vi "Get All Open Projects.vi"(8 "error in (no error)":errorcluster) -> (0 "error out":errorcluster, 1 "Names":string[](array[string]), 3 "Project refs out":refnum<vi>[](array[refnum]))   [LabVIEW 2019, in "Configuration Tool.lvlib"]
uses:
  Configuration Tool.lvlib
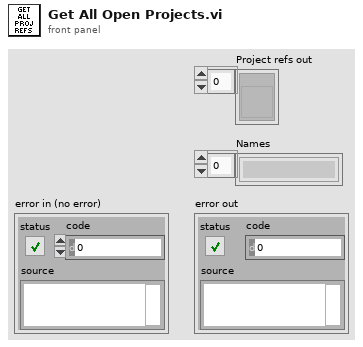
[diagram p1: front panel]
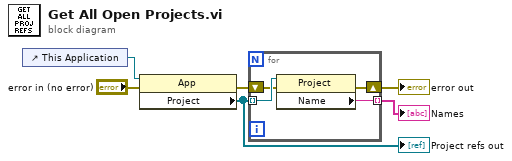
[diagram p0: block diagram]
diagram:
  n1 = control-ref of="This Application"() -> (w6:refnum<vi>)
  n2 = property class="App"(reference=w6, error in="error in (no error)") -> (error out=w2:errorcluster, "Project"=w4:refnum<vi>[])  [unwired: 1 out]
  "Project refs out" <- w4
  n3 = for {
    tunnel: w4 -> [w10] mode=indexing
    tunnel: [w9] -> w3 mode=indexing
    shift-right: [w7] -> w1
    shift-left: w2 -> [w8]
    n4 = property class="Project"(reference=w10, error in=w8) -> (error out=w7:errorcluster, "Name"=w9:string)  [unwired: 1 out]
  }
  "Names" <- w3
  "error out" <- w1
